vi "test starburst basic.vi"() -> ()   [LabVIEW 2015]
uses:
  connection/connection maintainer.lvclass
  client/connection client.lvclass/connection client.ctl
  message/communicator message.lvclass
  starburst/starburst.lvclass
  communicator/communicator.lvclass/communicator.ctl
  message/communicator message.lvclass/communicator message.ctl
  client/prepare client.vi
  server/prepare server.vi
  TCP client/TCP client.lvclass
  TCP/TCP server.lvclass
  communicator/communicator.lvclass
  <vilib>/ptbypt/NI_PtbyPt.lvlib
  manager/queue manager.lvclass
panel:
  out "Numeric 2":dbl
  out "data 3":variant
  out "ID 3":string
  out "data":variant
  out "ID":string
  out "Numeric":dbl
  in  "Boolean":bool
  in  "remake c":bool
  in  "CS 2":cluster{"ID":string, "data":string}
  in  "CS":cluster{"ID":string, "data":string}
  in  "S to C":bool
  in  "C to S":bool
  in  "exits":bool
  out "ClienT":timestamp
  out "servT":timestamp
  out "ClienQ":refnum<class "connection maintainer.lvclass">
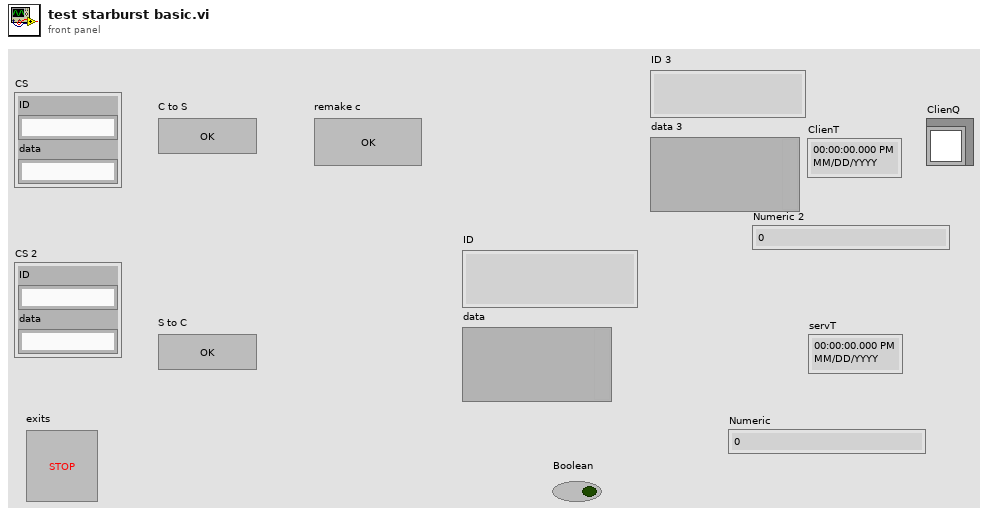
[diagram p1: front panel]
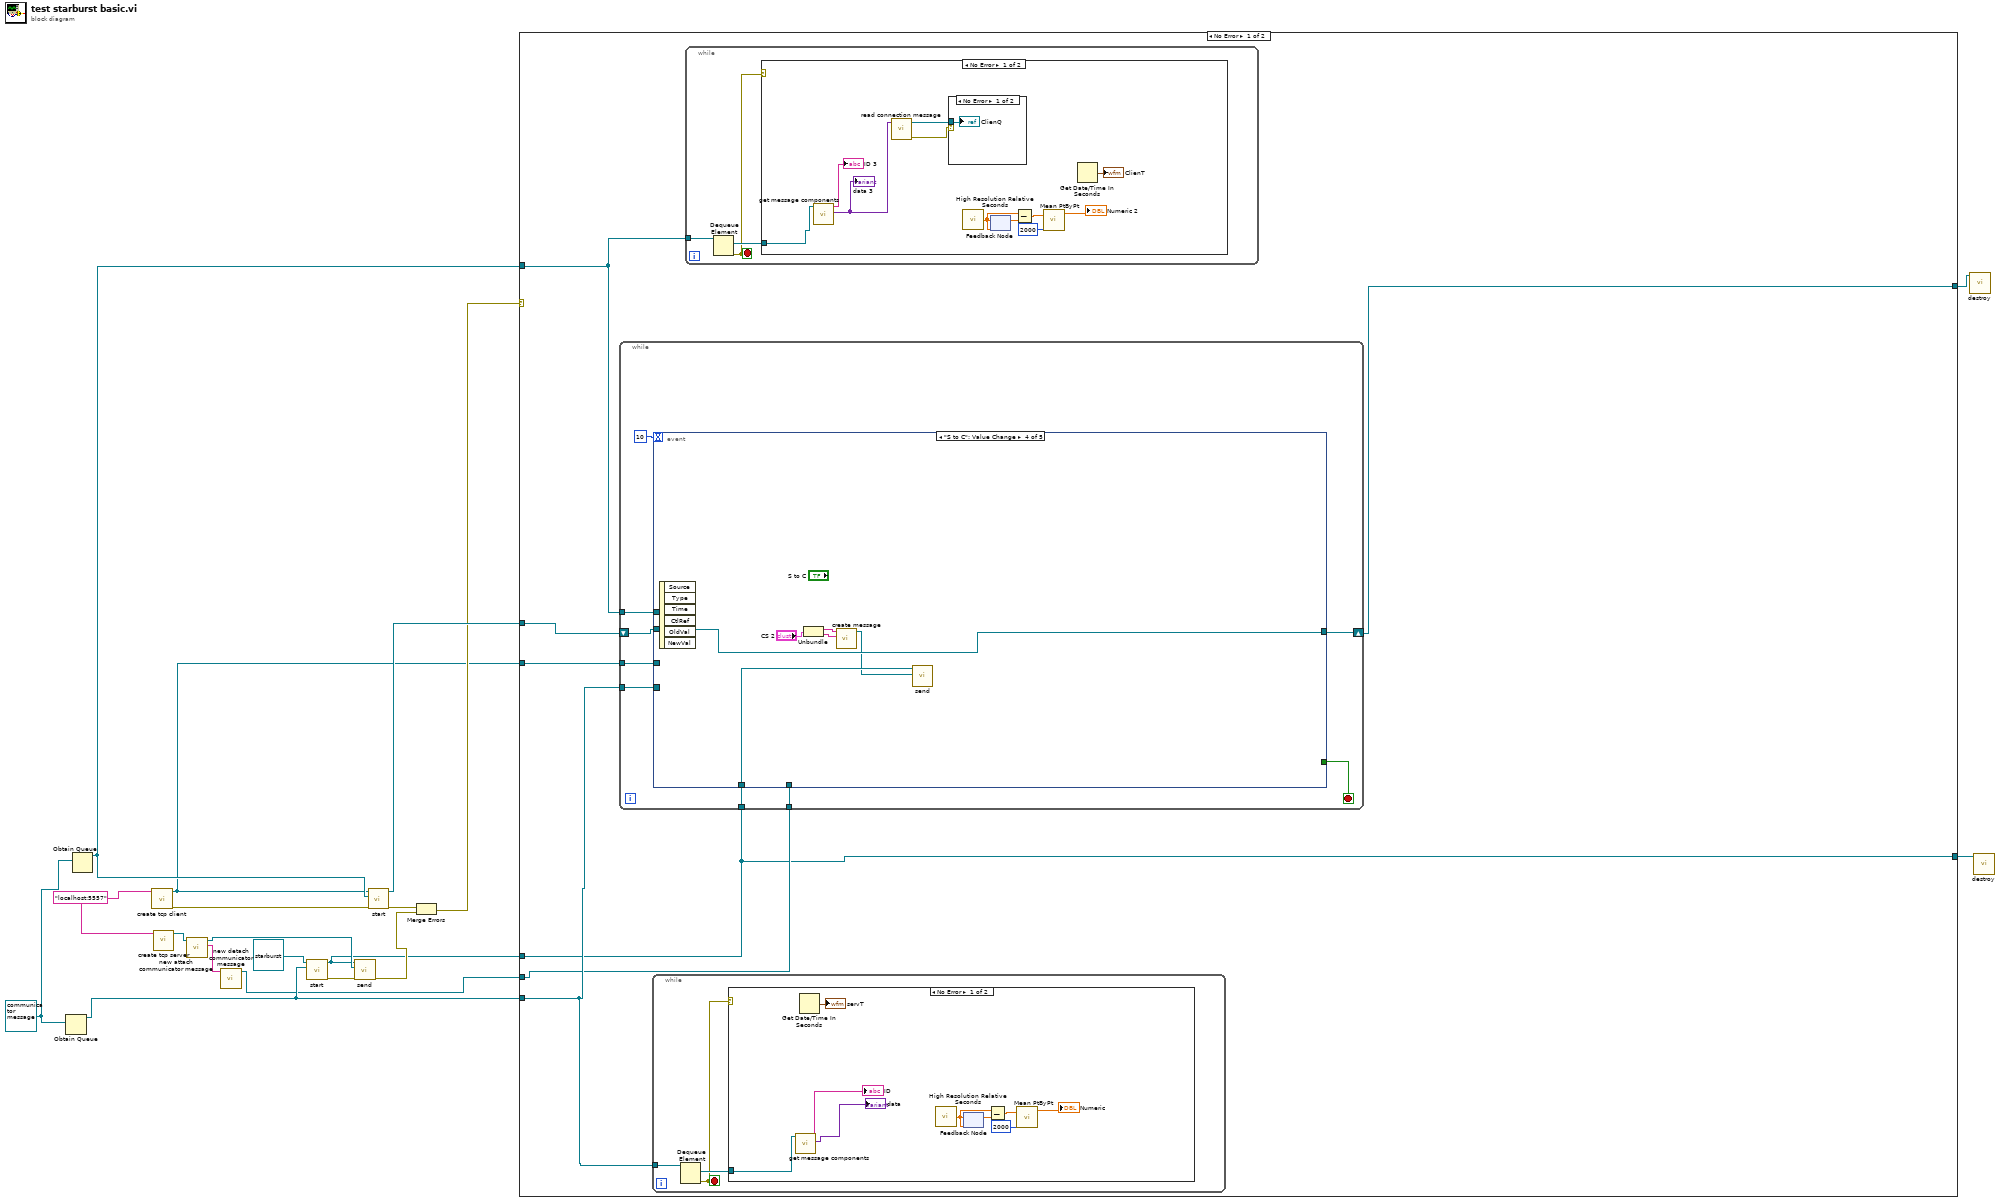
[diagram p0: block diagram]
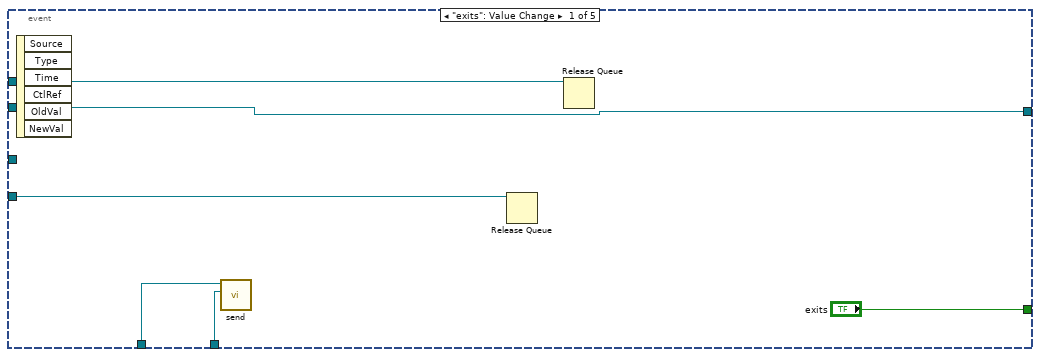
[diagram p2: hidden frame]
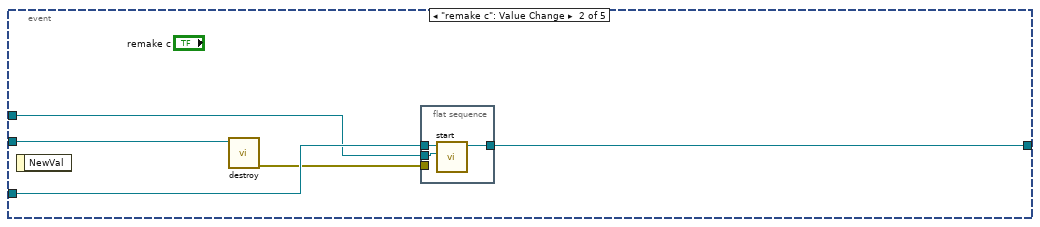
[diagram p3: hidden frame]
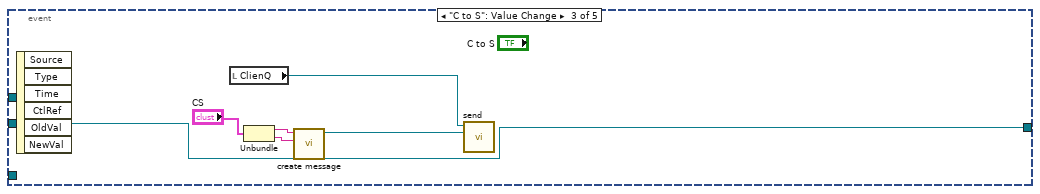
[diagram p4: hidden frame]
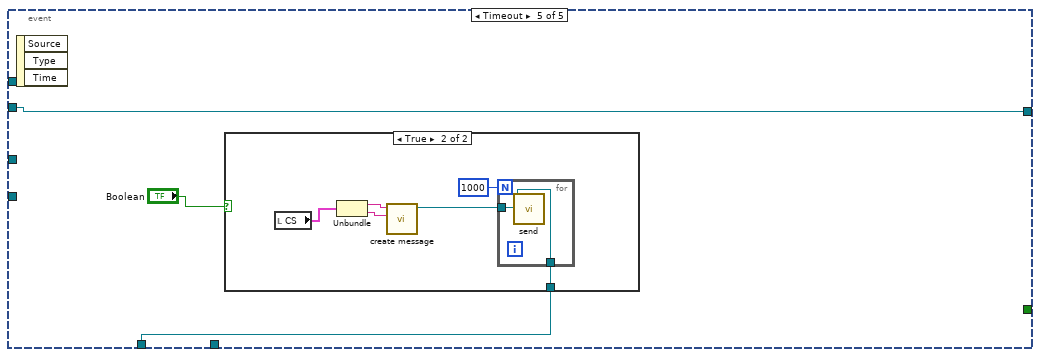
[diagram p5: hidden frame]
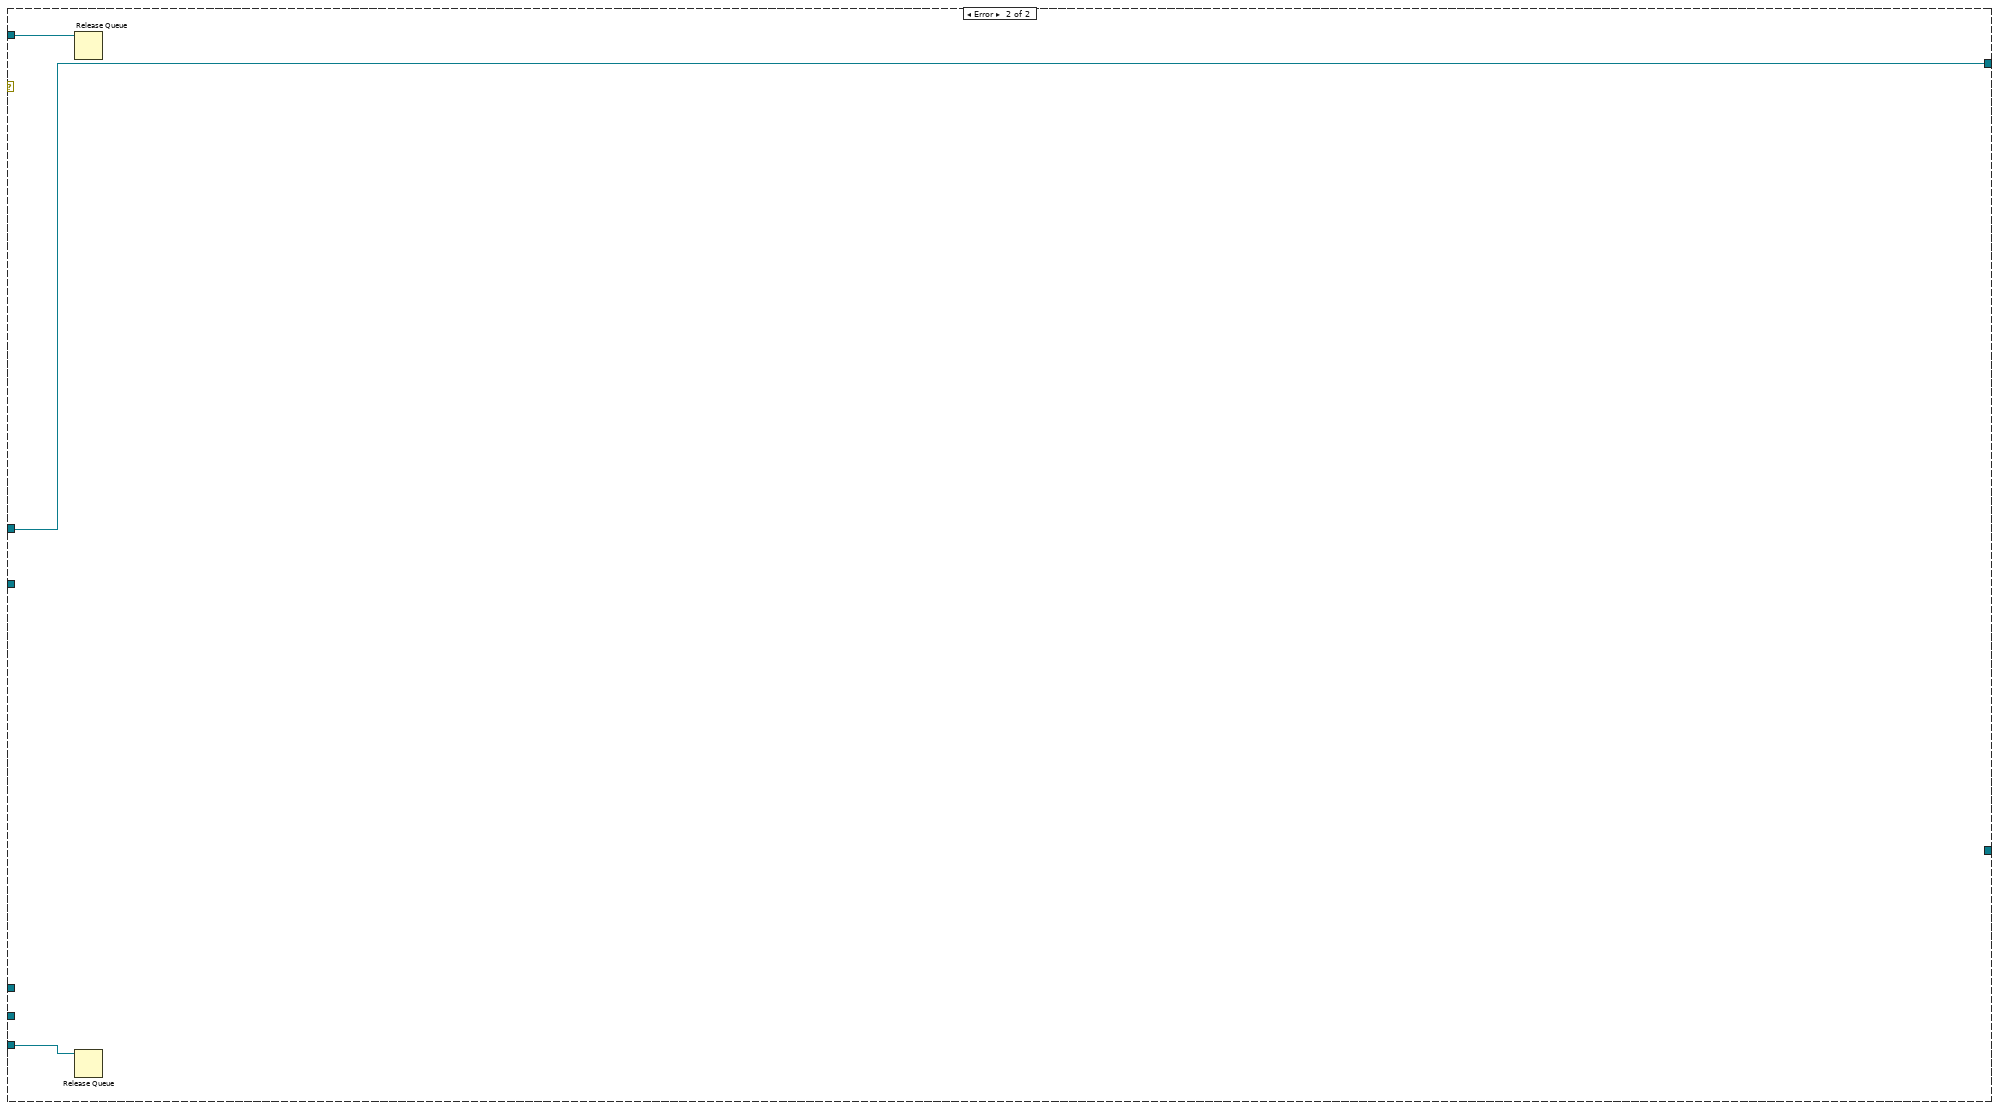
[diagram p10: hidden frame]
diagram:
  w11 = refnum<class "communicator message.lvclass"> refnum ("message")
  w15 = "localhost:5557" ("connection string")
  n1 = Obtain Queue(element data type=w11) -> (queue out=w9:refnum<queue>)  [unwired: 4 in, 2 out]
  n2 = Obtain Queue(element data type=w11) -> (queue out=w13:refnum<queue>)  [unwired: 4 in, 2 out]
  n3 = call "create tcp client.vi"("conn string"=w15) -> ("error out"=w18:errorcluster, "TCP client out"=w12:refnum<class "TCP client.lvclass">)  [unwired: 9 in]
  n4 = call "create tcp server.vi"("conn string"=w15) -> ("TCP server out"=w7:refnum<class "TCP server.lvclass">)  [unwired: 9 in, 1 out]
  n5 = call "new attach communicator message.vi"("comm"=w7) -> ("ID"=w6:string, "message"=w3:refnum<class "communicator message.lvclass">)  [unwired: 9 in]
  n6 = call "new detach communicator message.vi"("communicator to detach"=w6) -> ("message"=w5:refnum<class "communicator message.lvclass">)  [unwired: 10 in]
  n7 = call-dynamic "start.vi"("queue to parent"=w9, "communicator in"=refnum<class "starburst.lvclass"> refnum ("starburst")) -> ("error out"=w8:errorcluster, "communicator out"=w2:refnum<class "starburst.lvclass">)  [unwired: 8 in]
  n8 = call "send.vi"("error in"=w8, "element"=w3, "communicator in"=w2) -> ("error out"=w4:errorcluster)  [unwired: 8 in]
  n9 = call-dynamic "start.vi"("error in"=w18, "queue to parent"=w13, "communicator in"=w12) -> ("error out"=w16:errorcluster, "communicator out"=w17:refnum<class "TCP client.lvclass">)  [unwired: 7 in]
  n10 = Merge Errors(w16, w4) -> (w14:errorcluster)
  n11 = case shown="No Error" w14 {
    tunnel: [w22 w101] -> w19
    tunnel: w13 -> [w25 w102]
    tunnel: w17 -> [w24 w101]
    tunnel: w9 -> [w26 w100]
    tunnel: w12 -> [w23 _]
    tunnel: w5 -> [w21 _]
    tunnel: w2 -> [w20 _]
    tunnel: [w20 _] -> w1
    frame No Error {
      n12 = while {
        tunnel: w26 -> [w34]
        tunnel: w25 -> [w33]
        tunnel: w23 -> [w31]
        shift-right: [w30] -> w22
        shift-left: w24 -> [w32]
        tunnel: w20 -> [w28]
        tunnel: w21 -> [w27]
        stop <- w35 stop-if-true
        n13 = event shown="[3] \"S to C\": Value Change" {
          selector: _ -> [_ _ _ _ _]
          dyn-events: _ -> [_ _ _ _ _]
          timeout: 10 -> [_ _ _ _ _]
          tunnel: ["exits" _ _ _ _] -> w35
          tunnel: w34 -> [w40 _ _ _ _]
          tunnel: w33 -> [w39 w43 _ _ _]
          tunnel: w32 -> [w38 w46 w53 w61 w64]
          tunnel: w31 -> [_ w45 _ _ _]
          tunnel: [w38 w42 w53 w61 w64] -> w30
          tunnel: w28 -> [w37 _ _ w57 w62]
          tunnel: w27 -> [w36 _ _ _ _]
          event "exits": Value Change {
            n14 = event-data() -> ()  [unwired: 1 in, 6 out]
            n15 = call "send.vi"("element"=w36, "communicator in"=w37) -> ()  [unwired: 9 in, 1 out]
            n16 = Release Queue(queue=w40) -> ()  [unwired: 2 in, 3 out]
            n17 = Release Queue(queue=w39) -> ()  [unwired: 2 in, 3 out]
          }
          event "remake c": Value Change {
            n18 = event-data() -> ()  [unwired: 1 in, 1 out]
            n19 = call-dynamic "destroy.vi"("communicator in"=w46) -> ("error out"=w44:errorcluster)  [unwired: 10 in]
            n20 = flat-sequence {
              tunnel: w45 -> [w49]
              tunnel: w44 -> [_]
              tunnel: w43 -> [w48]
              tunnel: [w47] -> w42
              frame #0 {
                n21 = call-dynamic "start.vi"("queue to parent"=w48, "communicator in"=w49) -> ("communicator out"=w47:refnum<class "TCP client.lvclass">)  [unwired: 8 in, 1 out]
              }
            }
          }
          event "C to S": Value Change {
            n22 = event-data() -> ()  [unwired: 1 in, 6 out]
            n23 = local read "ClienQ"() -> (w55:refnum<class "connection maintainer.lvclass">)
            n24 = Unbundle("CS") -> ("ID"=w52:string, "data"=w51:string)
            n25 = call "create message.vi"("data"=w51, "ID"=w52) -> ("message"=w54:refnum<class "communicator message.lvclass">)  [unwired: 9 in]
            n26 = call "send.vi"("element"=w54, "communicator in"=w55) -> ()  [unwired: 9 in, 1 out]
          }
          event "S to C": Value Change {
            n27 = event-data() -> ()  [unwired: 1 in, 6 out]
            n28 = Unbundle("CS 2") -> ("ID"=w60:string, "data"=w59:string)
            n29 = call "create message.vi"("data"=w59, "ID"=w60) -> ("message"=w56:refnum<class "communicator message.lvclass">)  [unwired: 9 in]
            n30 = call "send.vi"("element"=w56, "communicator in"=w57) -> ()  [unwired: 9 in, 1 out]
          }
          event Timeout {
            n31 = event-data() -> ()  [unwired: 1 in, 3 out]
            n32 = case shown="True" "Boolean" {
              tunnel: w62 -> [_ w65]
              frame False {
              }
              frame True {
                n33 = local read "CS"() -> (w68:cluster{"ID":string, "data":string})
                n34 = Unbundle(w68) -> ("ID"=w70:string, "data"=w69:string)
                n35 = call "create message.vi"("data"=w69, "ID"=w70) -> ("message"=w67:refnum<class "communicator message.lvclass">)  [unwired: 9 in]
                n36 = for {
                  N: 1000 -> [_]
                  tunnel: w67 -> [w72]
                  tunnel: w65 -> [w71]
                  n37 = call "send.vi"("element"=w72, "communicator in"=w71) -> ()  [unwired: 9 in, 1 out]
                }
              }
            }
          }
        }
      }
      n38 = while {
        tunnel: w26 -> [w75]
        stop <- w73 stop-if-true
        n39 = Dequeue Element(queue=w75) -> (element=w74:refnum<class "communicator message.lvclass">, error out=w73:errorcluster)  [unwired: 2 in, 2 out]
        n40 = case shown="No Error" w73 {
          tunnel: w74 -> [w76 _]
          frame No Error {
            n41 = call "get message components.vi"("message"=w76) -> ("data"=→"data":variant, "ID"=→"ID":string)  [unwired: 9 in]
            n42 = Get Date/Time In Seconds() -> (seconds since 1Jan1904=→"servT":timestamp)
            n43 = call <vilib>:"High Resolution Relative Seconds.vi"() -> ("relative seconds"=w82:dbl)
            n44 = feedback-in #1(w82) -> ()
            n45 = feedback #1(w82) -> (w83:dbl)
            n46 = Subtract(x=w82, y=w83) -> (x-y=w81:dbl)
            n47 = call <vilib>:"Mean PtByPt.vi"("x"=w81, "sample length"=2000) -> ("mean"=→"Numeric":dbl)  [unwired: 2 in, 1 out]
          }
          frame Error {
          }
        }
      }
      n48 = while {
        tunnel: w25 -> [w87]
        stop <- w85 stop-if-true
        n49 = Dequeue Element(queue=w87) -> (element=w86:refnum<class "communicator message.lvclass">, error out=w85:errorcluster)  [unwired: 2 in, 2 out]
        n50 = case shown="No Error" w85 {
          tunnel: w86 -> [w94 _]
          frame No Error {
            n51 = call "get message components.vi"("message"=w94) -> ("data"=w93:variant, "ID"=→"ID 3":string)  [unwired: 9 in]
            "data 3" <- w93
            n52 = call "read connection message.vi"("data"=w93) -> ("error out"=w97:errorcluster, "conn"=w98:refnum<class "connection maintainer.lvclass">)  [unwired: 9 in]
            n53 = case shown="No Error" w97 {
              tunnel: w98 -> [w99 _]
              frame No Error {
                "ClienQ" <- w99
              }
              frame Error {
              }
            }
            n54 = call <vilib>:"High Resolution Relative Seconds.vi"() -> ("relative seconds"=w89:dbl)
            n55 = feedback #2(w89) -> (w88:dbl)
            n56 = feedback-in #2(w89) -> ()
            n57 = Subtract(x=w89, y=w88) -> (x-y=w90:dbl)
            n58 = call <vilib>:"Mean PtByPt.vi"("x"=w90, "sample length"=2000) -> ("mean"=→"Numeric 2":dbl)  [unwired: 2 in, 1 out]
            n59 = Get Date/Time In Seconds() -> (seconds since 1Jan1904=→"ClienT":timestamp)
          }
          frame Error {
          }
        }
      }
    }
    frame Error {
      n60 = Release Queue(queue=w102) -> ()  [unwired: 2 in, 3 out]
      n61 = Release Queue(queue=w100) -> ()  [unwired: 2 in, 3 out]
    }
  }
  n62 = call-dynamic "destroy.vi"("communicator in"=w19) -> ()  [unwired: 10 in, 1 out]
  n63 = call-dynamic "destroy.vi"("communicator in"=w1) -> ()  [unwired: 10 in, 1 out]
